vi "cg_fid_V1.2.vi"() -> ()   [LabVIEW 2011]
panel:
  in  "?":bool
  out "Start Indicator":bool
  in  "start chromat":bool
  in  "stop":bool
  in  "Voltage (AO)":dbl
  out "FID":cluster{"value":dbl}(graph)
  out "Temp History":cluster{"value":dbl}(graph)
  out "Integral":dbl
  out "Time (min)":dbl
  out "Counter":i32
  in  "Stop Time (min)":dbl=15.0
  out "Time has Elapsed":bool
  in  "Start Button":bool
  out "TCD":dbl(graph)
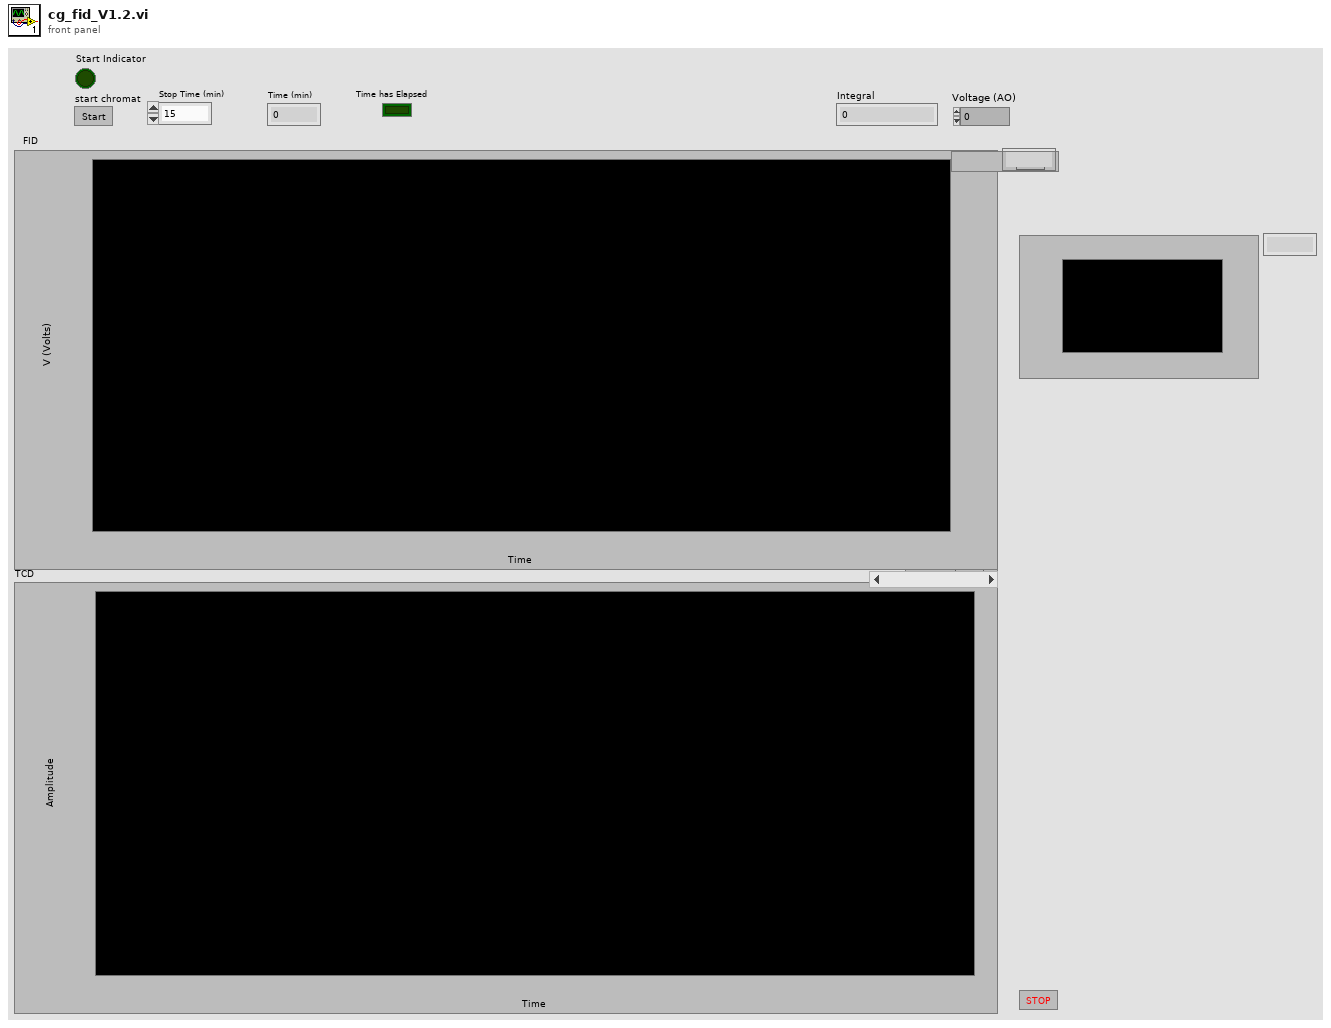
[diagram p1: front panel]
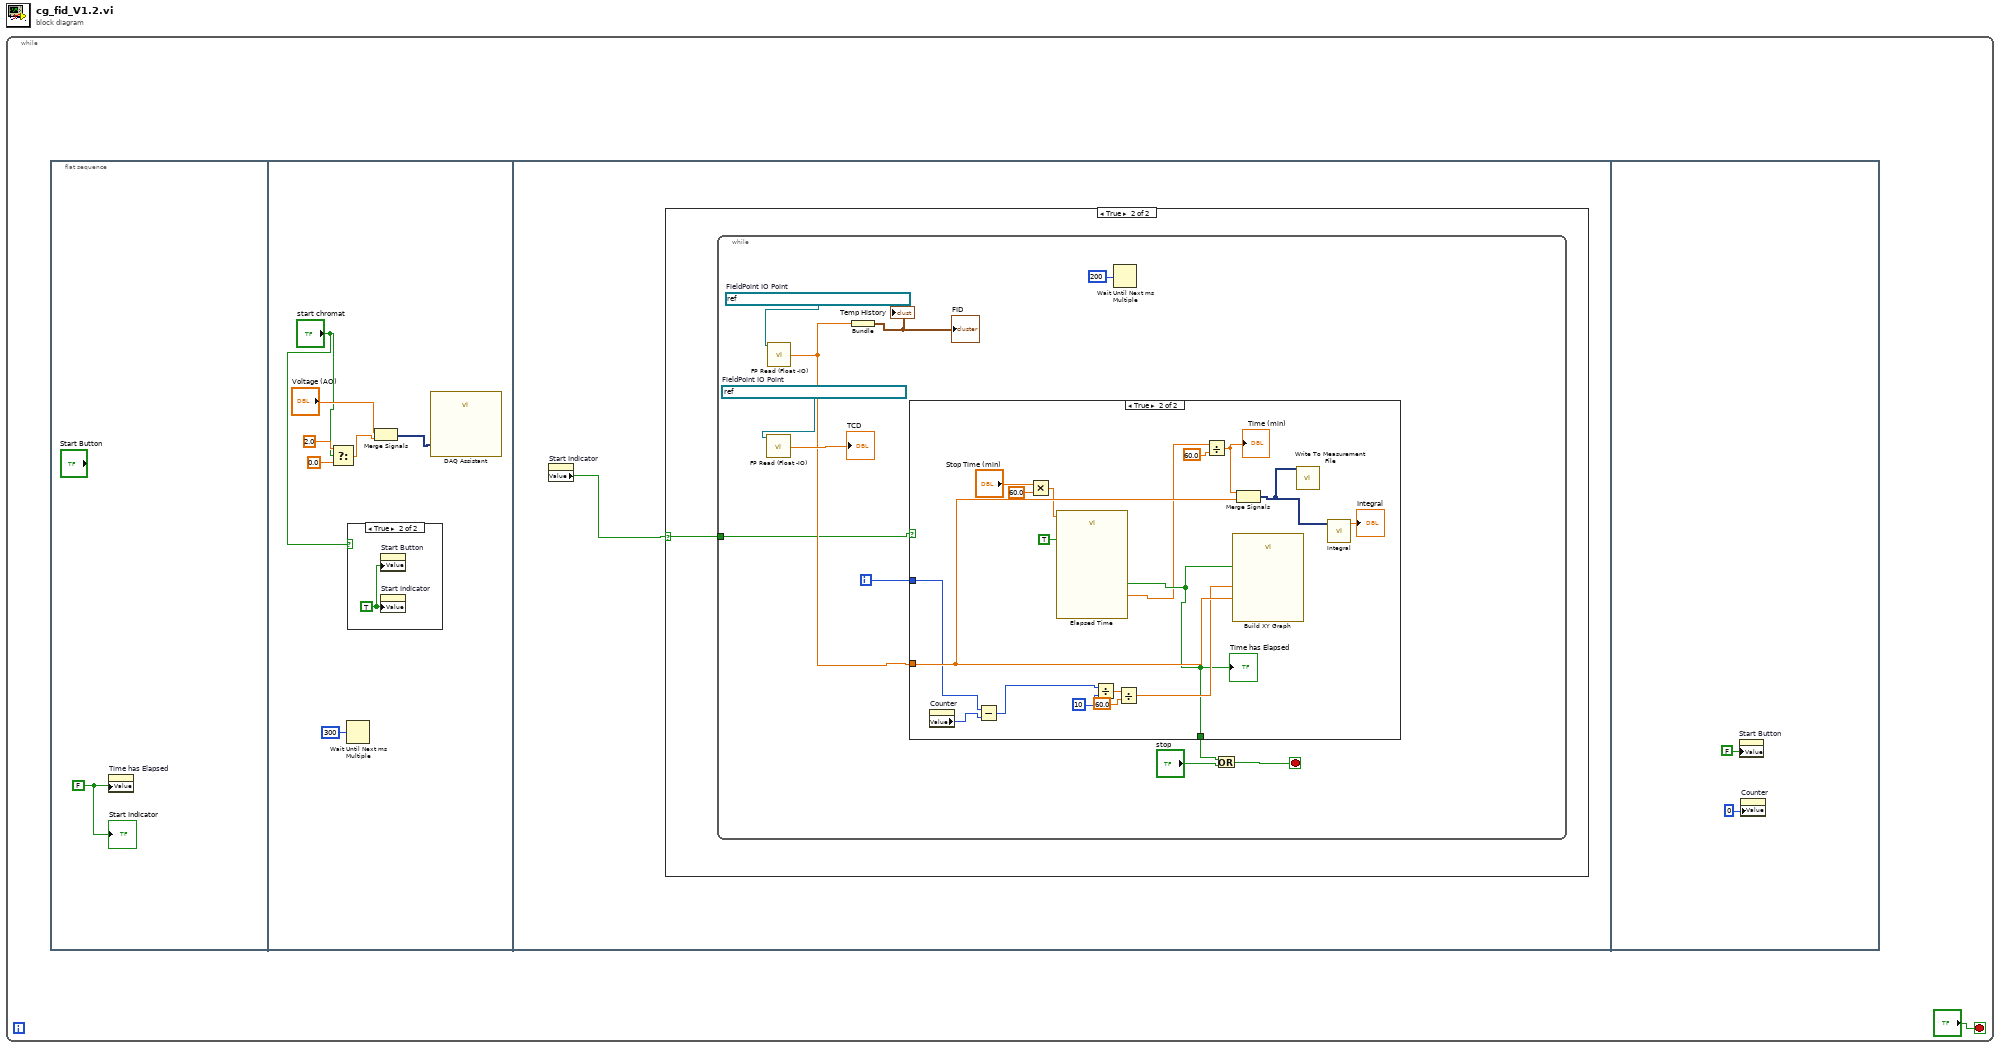
[diagram p0: block diagram]
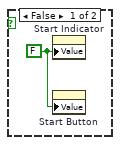
[diagram p2: hidden frame]
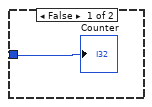
[diagram p4: hidden frame]
diagram:
  n1 = while {
    stop <- "?" stop-if-true
    n2 = flat-sequence {
      frame #0 {
        w2 = FALSE
        n3 = property on="Time has Elapsed" class="Bool (strict)"("Value"=w2) -> ()  [unwired: 2 in, 2 out]
        "Start Indicator" <- w2
      }
      frame #1 {
        n4 = Select(t=2.0, s="start chromat", f=0.0) -> (s? t:f=w3:dbl)
        n5 = Wait Until Next ms Multiple(millisecond multiple=u32 300) -> ()  [unwired: 1 out]
        n6 = case shown="True" "start chromat" {
          frame False {
            w10 = FALSE ("Start Button")
            n7 = property on="Start Indicator" class="Bool (strict)"("Value"=w10) -> ()  [unwired: 2 in, 2 out]
            n8 = property on="Start Button" class="Bool (strict)"("Value"=w10) -> ()  [unwired: 2 in, 2 out]
          }
          frame True {
            w11 = TRUE ("Start Button")
            n9 = property on="Start Button" class="Bool (strict)"("Value"=w11) -> ()  [unwired: 2 in, 2 out]
            n10 = property on="Start Indicator" class="Bool (strict)"("Value"=w11) -> ()  [unwired: 2 in, 2 out]
          }
        }
        n11 = Merge Signals("Voltage (AO)", w3) -> (w9:dynamicdata)
        n12 = call "DAQ Assistant"("data"=w9) -> ()  [unwired: 17 in, 2 out]
      }
      frame #2 {
        n13 = property on="Start Indicator" class="Bool (strict)"() -> ("Value"=w12:bool)  [unwired: 2 in, 2 out]
        n14 = case shown="True" w12 {
          selector: w12 -> [_ w13]
          frame False {
          }
          frame True {
            n15 = while {
              tunnel: w13 -> [w15]
              i -> [w20]
              stop <- w17 stop-if-true
              w23 = refnum<k21> "FieldPoint\\cfp2220\\cFP-AI-110 @4\\Channel 2"  # FieldPoint IO Point
              w24 = refnum<k21> "FieldPoint\\cfp2220\\cFP-AI-110 @4\\Channel 0"  # FieldPoint IO Point
              n16 = call <vilib>:"FP Read (Float -IO).vi"("FieldPoint IO Point In"=w23) -> ("value"=→"TCD":dbl)  [unwired: 11 in, 3 out]
              n17 = call <vilib>:"FP Read (Float -IO).vi"("FieldPoint IO Point In"=w24) -> ("value"=w18:dbl)  [unwired: 11 in, 3 out]
              n18 = Bundle("value"=w18) -> (→"Temp History" →"FID":cluster{"value":dbl})  [unwired: 1 out]
              n19 = case shown="True" w15 {
                tunnel: w18 -> [_ w43]
                tunnel: w20 -> [w25 w38]
                tunnel: [_ w29] -> w14
                frame False {
                  "Counter" <- w25
                }
                frame True {
                  n20 = property on="Counter" class="DigNum (strict)"() -> ("Value"=w37:i32)  [unwired: 2 in, 2 out]
                  n21 = Subtract(x=w38, y=w37) -> (x-y=w39:i32)
                  n22 = Multiply(x="Stop Time (min)", y=60.0) -> (x*y=w32:dbl)
                  n23 = call "Elapsed Time"("Time Target (s)"=w32, "Auto Reset"=TRUE) -> ("Elapsed Time (s)"=w28:dbl, "Time has Elapsed"=w29:bool)  [unwired: 10 in, 6 out]
                  "Time has Elapsed" <- w29
                  n24 = Divide(x=w39, y=10) -> (x/y=w41:dbl)
                  n25 = Divide(x=w41, y=60.0) -> (x/y=w36:dbl)
                  n26 = Divide(x=w28, y=60.0) -> (x/y=w27:dbl)
                  "Time (min)" <- w27
                  n27 = call "Build XY Graph"("Enable"=w29, "Y Input"=w43, "X Input"=w36) -> ()  [unwired: 2 in, 7 out]
                  n28 = Merge Signals(w27, w43) -> (w34:dynamicdata)
                  n29 = call "Write To Measurement File"("Signals"=w34) -> ()  [unwired: 16 in, 3 out]
                  n30 = call "Integral.vi"("Tested Signals"=w34) -> ("Integral"=→"Integral":dbl)  [unwired: 9 in, 1 out]
                }
              }
              n31 = Wait Until Next ms Multiple(millisecond multiple=u32 200) -> ()  [unwired: 1 out]
              n32 = Or(x=w14, y="stop") -> (x .or. y?=w17:bool)
            }
          }
        }
      }
      frame #3 {
        n33 = property on="Start Button" class="Bool (strict)"("Value"=FALSE ("Start Button")) -> ()  [unwired: 2 in, 2 out]
        n34 = property on="Counter" class="DigNum (strict)"("Value"=0 ("Numeric")) -> ()  [unwired: 2 in, 2 out]
      }
    }
  }
